vi "S2C_PCIe7841_Proc_DigitalReadLocal.vi"(8 "Error In":errorcluster, 9 "ExeRef":refnum<vi>, 11 "Q-Ref":refnum<queue>) -> (0 "Error Out":errorcluster, 3 "Command":string)   [LabVIEW 2015]
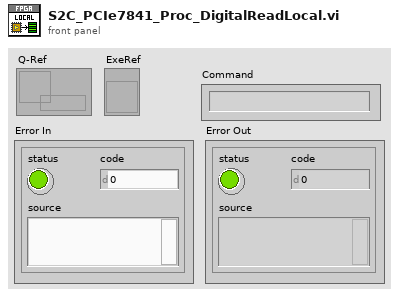
[diagram p1: front panel]
types:
  T1 = cluster{"Caller-Q":refnum<queue>, "Command":string, "Return":string, "Data":variant, "Timeout":dbl}
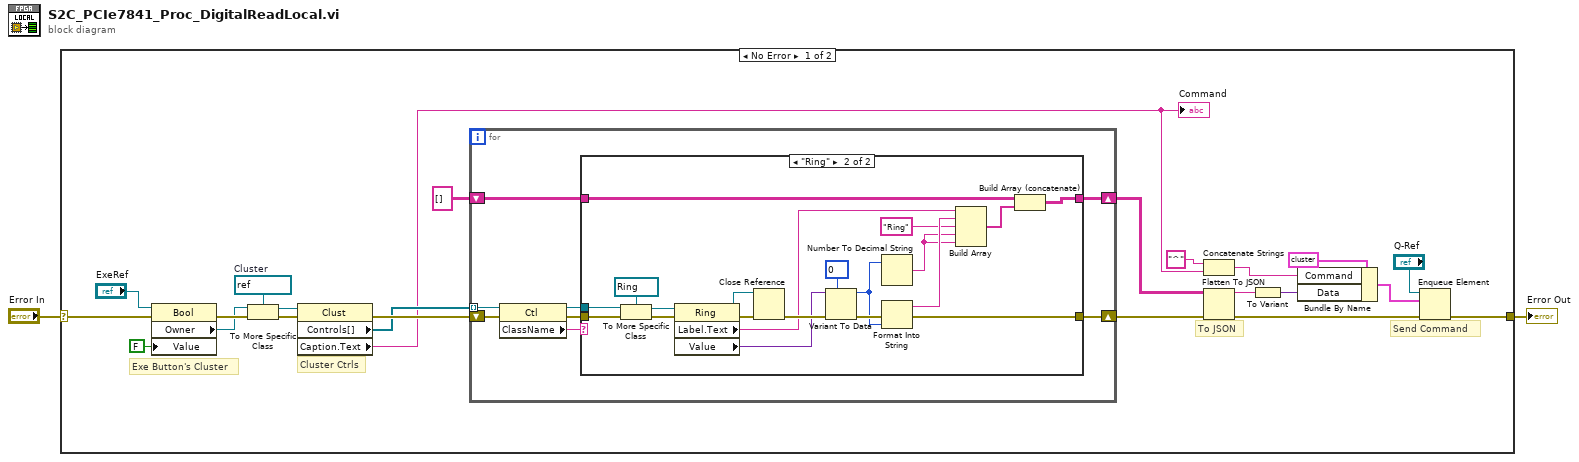
[diagram p0: block diagram]
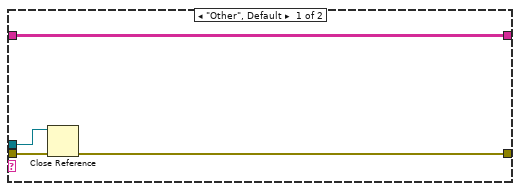
[diagram p2: hidden frame]
diagram:
  n1 = case shown="No Error" "Error In" {
    selector: "Error In" -> [w17 w58]
    tunnel: [w15 w58] -> w1
    frame No Error {
      w22 = refnum<vi> refnum  # Cluster
      # "Send Command"
      # "To JSON"
      # "Cluster Ctrls"
      # "Exe Button's Cluster"
      n2 = property class="Bool"(reference="ExeRef", error in=w17, "Value"=FALSE) -> (error out=w24:errorcluster, "Owner"=w23:refnum<vi>)  [unwired: 1 out]
      n3 = To More Specific Class(target class=w22, reference=w23, error in=w24) -> (specific class reference=w20:refnum<vi>, error out=w21:errorcluster)
      n4 = property class="Clust"(reference=w20, error in=w21) -> (error out=w19:errorcluster, "Controls[]"=w18:refnum<vi>[], "Caption.Text"=w10:string)  [unwired: 1 out]
      "Command" <- w10
      n5 = for {
        tunnel: w18 -> [w32] mode=indexing
        shift-right: [w28] -> w16
        shift-left: w19 -> [w33]
        shift-right: [w26] -> w4
        shift-left: string[][] [] ("Array - String") -> [w27]
        n6 = property class="Ctl"(reference=w32, error in=w33) -> (reference out=w29:refnum<vi>, error out=w31:errorcluster, "ClassName"=w30:string)
        n7 = case shown="\"Ring\"" w30 {
          tunnel: [w37 w48] -> w28
          tunnel: w31 -> [w36 w42]
          tunnel: w29 -> [w35 w41]
          tunnel: w27 -> [w34 w40]
          tunnel: [w34 w38] -> w26
          frame "Other", Default {
            n8 = Close Reference(reference=w35, error in (no error)=w36) -> (error out=w37:errorcluster)
          }
          frame "Ring" {
            w43 = u16 0 items=[""]
            n9 = To More Specific Class(target class=refnum<vi> refnum ("reference"), reference=w41, error in=w42) -> (specific class reference=w56:refnum<vi>, error out=w57:errorcluster)
            n10 = property class="Ring"(reference=w56, error in=w57) -> (reference out=w54:refnum<vi>, error out=w55:errorcluster, "Label.Text"=w50:string, "Value"=w51:variant)
            n11 = Close Reference(reference=w54, error in (no error)=w55) -> (error out=w52:errorcluster)
            n12 = Variant To Data(error in=w52, type=w43, Variant=w51) -> (data=w47:u16, error out=w49:errorcluster)
            n13 = Number To Decimal String(number=w47) -> (decimal integer string=w44:string)  [unwired: 1 in]
            n14 = Format Into String(error in=w49, w47) -> (resulting string=w46:string, error out=w48:errorcluster)  [unwired: 2 in]
            n15 = Build Array(w50, w46, "Ring" ("element"), w44, w44) -> (w39:string[])
            n16 = Build Array (concatenate)(w40, w39) -> (w38:string[][])
          }
        }
      }
      n17 = Concatenate Strings("^" ("string"), w10) -> (w11:string)
      n18 = Flatten To JSON(anything=w4, error in (no error)=w16) -> (JSON string=w13:string, 11:w14:errorcluster)  [unwired: 1 in]
      n19 = To Variant(anything=w13) -> (Variant=w8:variant)
      n20 = Bundle By Name(cluster=T1 {"Caller-Q"=refnum, "Command"="", "Return"="None", "Data"=variant, "Timeout"=10.0} ("element"), "Command"=w11, "Data"=w8) -> (w7:T1)
      n21 = Enqueue Element(queue="Q-Ref", element=w7, error in (no error)=w14) -> (error out=w15:errorcluster)  [unwired: 1 in, 2 out]
    }
    frame Error {
    }
  }
  "Error Out" <- w1
